vi "getTemp.vi"(0 "Handle In":i32, 1 "AIN Range":u16(ring) items=["LJ_rgBIP10V", "LJ_rgBIP1V", "LJ_rgBIPP1V", "LJ_rgBIPP01V"], 5 "+Channel":u16, 7 "Thermocouple Type":u16(ring) items=["B", "E", "J", "K", "N", "R", "S", "T"], 9 "-Channel":u16, 11 "error in":errorcluster, 12 "Offset Voltages":dbl format="%.6f") -> (3 "Cold Junction\nTemperature (Deg C)":dbl format="%.2f", 4 "Raw Readings":dbl format="%.6f", 6 "Temperature (Deg F)":dbl format="%.2f", 8 "Temperature (Deg C)":dbl format="%.2f", 10 "Temperature (Kelvin)":dbl format="%.2f", 15 "error out":errorcluster)   [LabVIEW 2021]
panel:
  # "inputs"
  # "outputs"
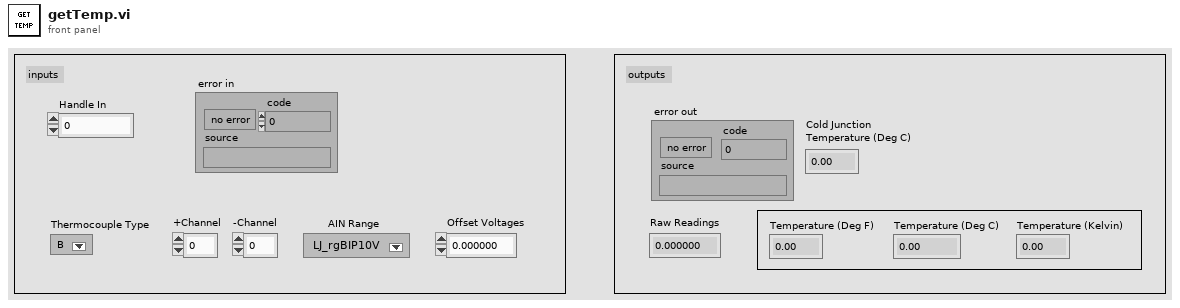
[diagram p1: front panel]
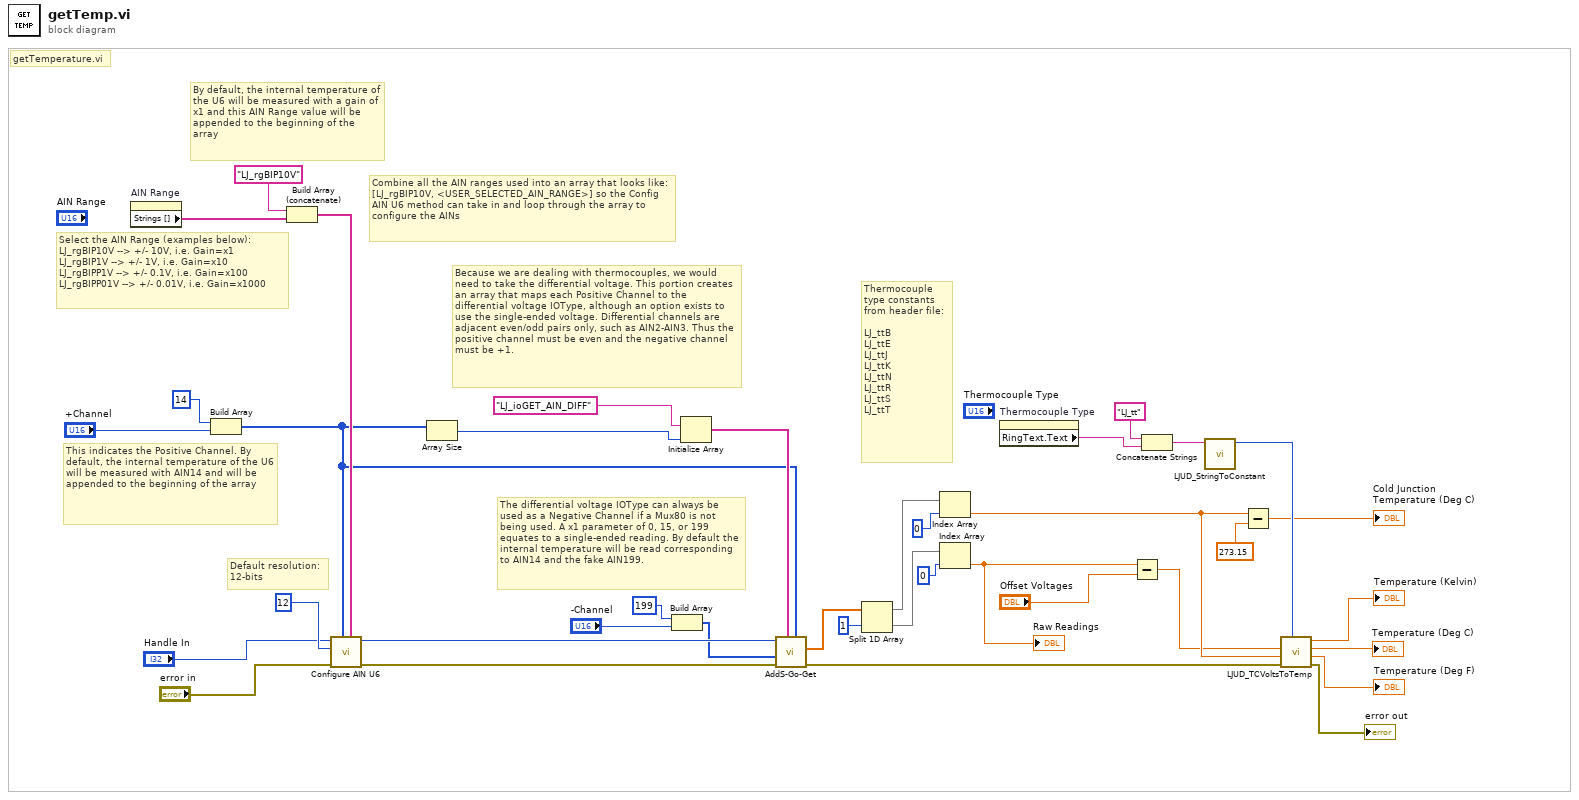
[diagram p0: block diagram]
diagram:
  # "getTemperature.vi"
  # "Thermocouple\ntype constants\nfrom header file:\n\nLJ_ttB\nLJ_ttE\nLJ_ttJ\nLJ_ttK\nLJ_ttN\nLJ_ttR\nLJ_ttS\nLJ_ttT"
  # "The differential voltage IOType can always be used as a Negative Channel if a Mux80 is not being used. A x1 parameter of 0, 15, or 199 equates to a single-ended reading. By default the internal temperature will be read corresponding to AIN14 and the fake AIN199."
  # "Because we are dealing with thermocouples, we would need to take the differential voltage. This portion creates an array that maps each Positive Channel to the differential voltage IOType, although an option exists to use the single-ended voltage. Differential channels are adjacent even/odd pairs only, such as AIN2-AIN3. Thus the positive channel must be even and the negative channel must be +1."
  # "This indicates the Positive Channel. By default, the internal temperature of the U6 will be measured with AIN14 and will be appended to the beginning of the array"
  # "Combine all the AIN ranges used into an array that looks like: [LJ_rgBIP10V, <USER_SELECTED_AIN_RANGE>] so the Config AIN U6 method can take in and loop through the array to configure the AINs"
  # "By default, the internal temperature of the U6 will be measured with a gain of x1 and this AIN Range value will be appended to the beginning of the array"
  # "Default resolution:\n12-bits"
  # "Select the AIN Range (examples below):\nLJ_rgBIP10V --> +/- 10V, i.e. Gain=x1\nLJ_rgBIP1V --> +/- 1V, i.e. Gain=x10\nLJ_rgBIPP1V --> +/- 0.1V, i.e. Gain=x100\nLJ_rgBIPP01V --> +/- 0.01V, i.e. Gain=x1000"
  n1 = property on="AIN Range" class="Ring (strict)"() -> ("Strings []"=w12:string[])  [unwired: 2 in, 2 out]
  n2 = Build Array(u16 14 ("element"), "+Channel") -> (w16:u16[])
  n3 = Build Array (concatenate)("LJ_rgBIP10V" ("DeviceType"), w12) -> (w33:string[])
  n4 = call <vilib>:"Configure AIN U6.vi"("Ranges"=w33, "Positive Channels"=w16, "error in"="error in", "Resolution"=12, "Handle In"="Handle In") -> ("error out"=w36:errorcluster, "Handle Out"=w35:i32)  [unwired: 5 in]
  n5 = Array Size(array=w16) -> (size(s)=w30:i32)
  n6 = Build Array(u16 199 ("element"), "-Channel") -> (w28:u16[])
  n7 = Initialize Array("LJ_ioGET_AIN_DIFF" ("IOType"), w30) -> (w37:string[])
  n8 = call <vilib>:"AddS-Go-Get.vi"("Channels"=w16, "IOTypes"=w37, "error in"=w36, "x1"=w28, "Handle In"=w35) -> ("error out"=w13:errorcluster, "Values Read"=w22:dbl[])  [unwired: 4 in, 1 out]
  n9 = Split 1D Array(array=w22, index=1) -> (first subarray=w26:dbl[], second subarray=w15:dbl[])
  n10 = Index Array(array=w26, index=0 ("Index")) -> (element=w10:dbl)
  n11 = Index Array(array=w15, index=0) -> (element=w6:dbl)
  "Raw Readings" <- w6
  n12 = property on="Thermocouple Type" class="Ring (strict)"() -> ("RingText.Text"=w20:string)  [unwired: 2 in, 2 out]
  n13 = Subtract(x=w6, y="Offset Voltages") -> (x-y=w9:dbl)
  n14 = Concatenate Strings("LJ_tt" ("string"), w20) -> (w19:string)
  n15 = call <vilib>:"LJUD_StringToConstant.vi"("String"=w19) -> ("Constant Number"=w14:i32)  [unwired: 9 in, 1 out]
  n16 = Subtract(x=w10, y=273.15) -> (x-y=→"Cold Junction\nTemperature (Deg C)":dbl)
  n17 = call <vilib>:"LJUD_TCVoltsToTemp.vi"("TCType"=w14, "error in"=w13, "CJTempK"=w10, "TCVolts"=w9) -> ("error out"=→"error out":errorcluster, "TCTempF"=→"Temperature (Deg F)":dbl, "TCTempC"=→"Temperature (Deg C)":dbl, "TCTempK"=→"Temperature (Kelvin)":dbl)  [unwired: 4 in]
